vi "DestroySession.vi"(8 "error in (no error)":errorcluster, 11 "session id in":i32) -> (0 "error out":errorcluster, 2 "return":i32)   [LabVIEW 2017, in "libonnx_wrapper.lvlib"]
doc: "/**\n * @brief Полностью удалить сессию (очистить память и освободить ID)\n * \n * Эта функция полностью уничтожает сессию: освобождает память модели,\n * удаляет метаданные, освобождает путь к файлу и удаляет SessionID из хранилища.\n * После вызова этой функции SessionID становится невалидным.\n * \n * @param sessionId [IN] ID сессии для удаления\n * \n * @return int32: 0 при успешном удалении\n * @return int32: -1 если сессия не найдена\n * \n * @note Обязательно вызывать при завершении работы с моделью\n * @note После вызова SessionID нельзя использовать повторно\n */\nint DestroySession(int sessionId);"
uses:
  libonnx_wrapper.lvlib
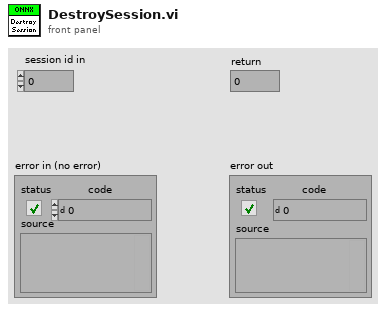
[diagram p1: front panel]
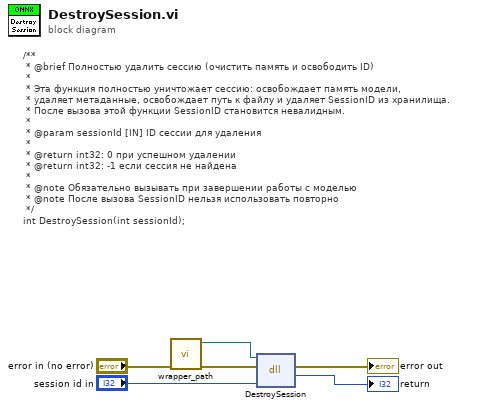
[diagram p0: block diagram]
diagram:
  # "/**\n * @brief Полностью удалить сессию (очистить память и освободить ID)\n * \n * Эта функция полностью уничтожает сессию: освобождает память модели,\n * удаляет метаданные, освобождает путь к файлу и удаляет SessionID из хранилища.\n * После вызова этой функции SessionID становится невалидным.\n * \n * @param sessionId [IN] ID сессии для удаления\n * \n * @return int32: 0 при успешном удалении\n * @return int32: -1 если сессия не найдена\n * \n * @note Обязательно вызывать при завершении работы с моделью\n * @note После вызова SessionID нельзя использовать повторно\n */\nint DestroySession(int sessionId);"
  n1 = call "wrapper_path.vi"("error in (no error)"="error in (no error)") -> ("error out"=w4:errorcluster, "wrapper path"=w3:path)  [unwired: 9 in]
  n2 = dll-call lib="home/ivan/LabVIEWData/ONNX/Test/libonnx_wrapper/unix64/libonnx_wrapper.so" fn="DestroySession"(path in=w3, error in=w4, "sessionId"="session id in") -> (error out=→"error out":errorcluster, "return type"=→"return":i32)  [unwired: 2 in, 1 out]
